vi "Vector_arrow.vi"(10 "vector":cluster{"length":dbl, "angle":dbl}, 11 "tip":cluster{dbl, dbl}) -> (3 "(x,y)":cluster{dbl, dbl}[](array[cluster]))   [LabVIEW 2024]
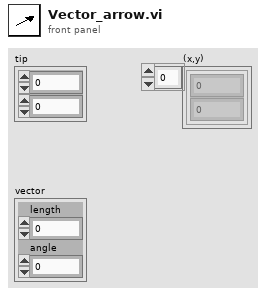
[diagram p1: front panel]
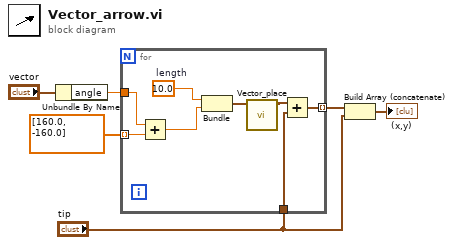
[diagram p0: block diagram]
diagram:
  n1 = Unbundle By Name("vector") -> ("angle"=w2:dbl)
  n2 = for {
    tunnel: "tip" -> [w7]
    tunnel: dbl[] [160.0, -160.0] -> [w11] mode=indexing
    tunnel: [w10] -> w4 mode=indexing
    tunnel: w2 -> [w9]
    w12 = 10.0  # length
    n3 = Add(x=w9, y=w11) -> (x+y=w14:dbl)
    n4 = Bundle("length"=w12, w14) -> (w13:cluster{"length":dbl, dbl})  [unwired: 1 in]
    n5 = call "Vector_place.vi"("vector"=w13) -> ("x,y"=w8:cluster{dbl, dbl})  [unwired: 10 in]
    n6 = Add(x=w8, y=w7) -> (x+y=w10:cluster{dbl, dbl})
  }
  n7 = Build Array (concatenate)(w4, "tip") -> (→"(x,y)":cluster{dbl, dbl}[])
